vi "test_libssh2_session_blocking.vi"() -> ()   [LabVIEW 2017, in "unit_tests.lvlib"]
uses:
  unit_tests.lvlib
  libssh2/libssh2_init_default.vi
  libssh2/libssh2_session_init_ex.vi
  libssh2/libssh2.lvlib
  <vilib>/PNR/Transparent Assertions/Transparent Assertions/Transparent Assertions.lvlib
panel:
  out "error out":errorcluster
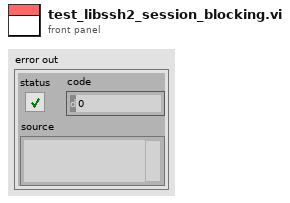
[diagram p1: front panel]
types:
  T1 = typedef "libssh2.lvlib/Session Refnum.ctl" = refnum<k1>
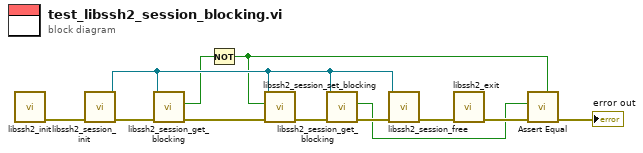
[diagram p0: block diagram]
diagram:
  n1 = call-poly "libssh2_init.vi"() -> ("error out"=w11:errorcluster)  [unwired: 11 in]
  n2 = call "libssh2_session_init.vi"("error in (no error)"=w11) -> ("error out"=w5:errorcluster, "session"=w4:T1)  [unwired: 9 in]
  n3 = call "libssh2_session_get_blocking.vi"("error in (no error)"=w5, "session"=w4) -> ("error out"=w6:errorcluster, "blocking"=w3:bool)  [unwired: 8 in]
  n4 = Not(x=w3) -> (.not. x?=w1:bool)
  n5 = call "libssh2_session_set_blocking.vi"("error in (no error)"=w6, "blocking"=w1, "session"=w4) -> ("error out"=w9:errorcluster)  [unwired: 8 in]
  n6 = call "libssh2_session_get_blocking.vi"("error in (no error)"=w9, "session"=w4) -> ("error out"=w7:errorcluster, "blocking"=w2:bool)  [unwired: 8 in]
  n7 = call "libssh2_session_free.vi"("error in (no error)"=w7, "session"=w4) -> ("error out"=w10:errorcluster)  [unwired: 9 in]
  n8 = call "libssh2_exit.vi"("error in (no error)"=w10) -> ("error out"=w8:errorcluster)  [unwired: 10 in]
  n9 = call <vilib>:"Assert Equal.vi"("Expected"=w1, "error in (no error)"=w8, "Actual"=w2) -> ("error out"=→"error out":errorcluster)  [unwired: 8 in]
